vi "PBLV_Interface.vi"() -> ()   [LabVIEW 2013]
uses:
  <vilib>/Utility/error.llb/DialogTypeEnum.ctl
panel:
  in  "board_num":i32
  in  "change board":bool
  in  "# of Instructions":u32=4
  in  "Path to spinapi.dll":path=path "C:/SpinCore/SpinAPI/lib32/spinapi.dll"
  in  "start/restart":bool
  in  "load":bool
  in  "stop":bool
  in  "clock_freq (MHz)":dbl=100.0
  in  "Instructions":T1(array[cluster])=[{"Instruct Data"=0, "Op Code"=0, "Flags"=[FALSE, FALSE, FALSE, TRUE, FALSE, FALSE, FALSE, FALSE, FALSE, FALSE, FALSE, FALSE, FALSE, FALSE, FALSE, FALSE, FALSE, FALSE, FALSE, FALSE, FALSE, FALSE, FALSE, FALSE], "Comments"="", "Time (s)"=3e-05}, {"Instruct Data"=0, "Op Code"=0, "Flags"=[FALSE, TRUE, TRUE, FALSE, FALSE, FALSE, FALSE, FALSE, FALSE, FALSE, FALSE, FALSE, FALSE, FALSE, FALSE, FALSE, FALSE, FALSE, FALSE, FALSE, FALSE, FALSE, FALSE, FALSE], "Comments"="", "Time (s)"=0.5}, {"Instruct Data"=0, "Op Code"=0, "Flags"=[FALSE, FALSE, FALSE, TRUE, FALSE, FALSE, FALSE, FALSE, FALSE, FALSE, FALSE, FALSE, FALSE, FALSE, FALSE, FALSE, FALSE, FALSE, FALSE, FALSE, FALSE, FALSE, FALSE, FALSE], "Comments"="", "Time (s)"=3e-05}, {"Instruct Data"=0, "Op Code"=6, "Flags"=[FALSE, TRUE, TRUE, FALSE, FALSE, FALSE, FALSE, FALSE, FALSE, FALSE, FALSE, FALSE, FALSE, FALSE, FALSE, FALSE, FALSE, FALSE, FALSE, FALSE, FALSE, FALSE, FALSE, FALSE], "Comments"="", "Time (s)"=0.5}, {"Instruct Data"=0, "Op Code"=0, "Flags"=[TRUE, TRUE, TRUE, FALSE, FALSE, FALSE, FALSE, FALSE, FALSE, FALSE, FALSE, FALSE, FALSE, FALSE, FALSE, FALSE, FALSE, FALSE, FALSE, FALSE, FALSE, FALSE, FALSE, FALSE], "Comments"="", "Time (s)"=1.0}, {"Instruct Data"=0, "Op Code"=6, "Flags"=[FALSE, TRUE, TRUE, FALSE, FALSE, FALSE, FALSE, FALSE, FALSE, FALSE, FALSE, FALSE, FALSE, FALSE, FALSE, FALSE, FALSE, FALSE, FALSE, FALSE, FALSE, FALSE, FALSE, FALSE], "Comments"="", "Time (s)"=0.0015}] {"Time (s)" format="%.3p"; "Op Code" items=["Continue", "Stop", "Loop", "End Loop", "JSR", "RTS", "Branch", "Long Delay", "Wait"]}
  # "LabVIEW PulseBlaster Extension\nPulseBlaster Interface\nSpinCore Technologies, Inc.\nwww.spincore.com"
  # "Caution:    \n            After pressing STOP,\n            all output bits may \nmaintain their final state."
  # "1"
  # "2"
  # "3"
  # "4"
  # "5"
  # "6"
  # "7"
  # "8"
  # "9"
  # "10"
  # "11"
  # "12"
  # "13"
  # "14"
  # "15"
  # "16"
  # "17"
  # "18"
  # "19"
  # "20"
  # "21"
  # "22"
  # "23"
  # "24"
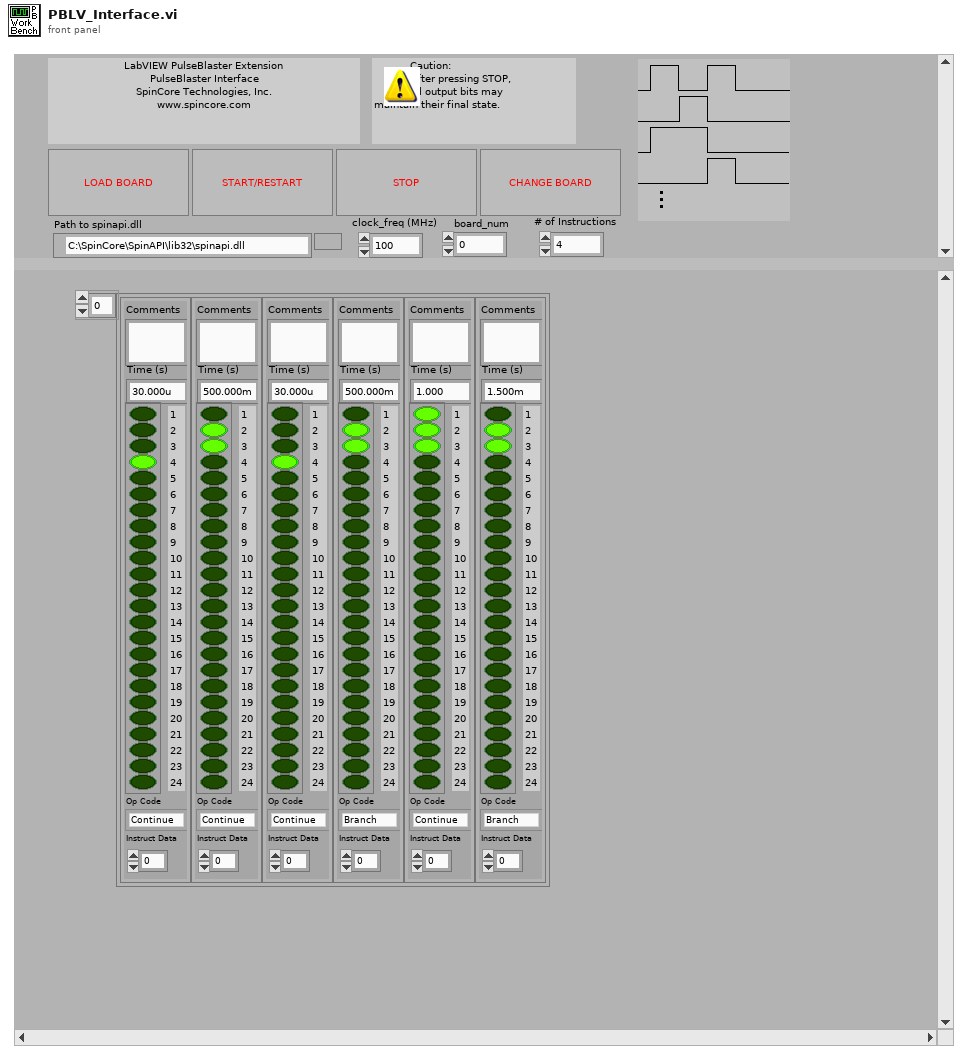
[diagram p1: front panel]
types:
  T1 = cluster{"Instruct Data":i32, "Op Code":i32, "Flags":bool[], "Comments":string, "Time (s)":dbl}[]
  T2 = typedef "DialogTypeEnum.ctl" = enum16{"no dialog", "OK message", "continue or stop message", "auto error handling dialog", "OK message + warnings", "continue/stop + warnings"}
  T3 = enum16{"Pulse Program", "Frequency Registers", "TX Phase Registers", "RX Phase Registers"}
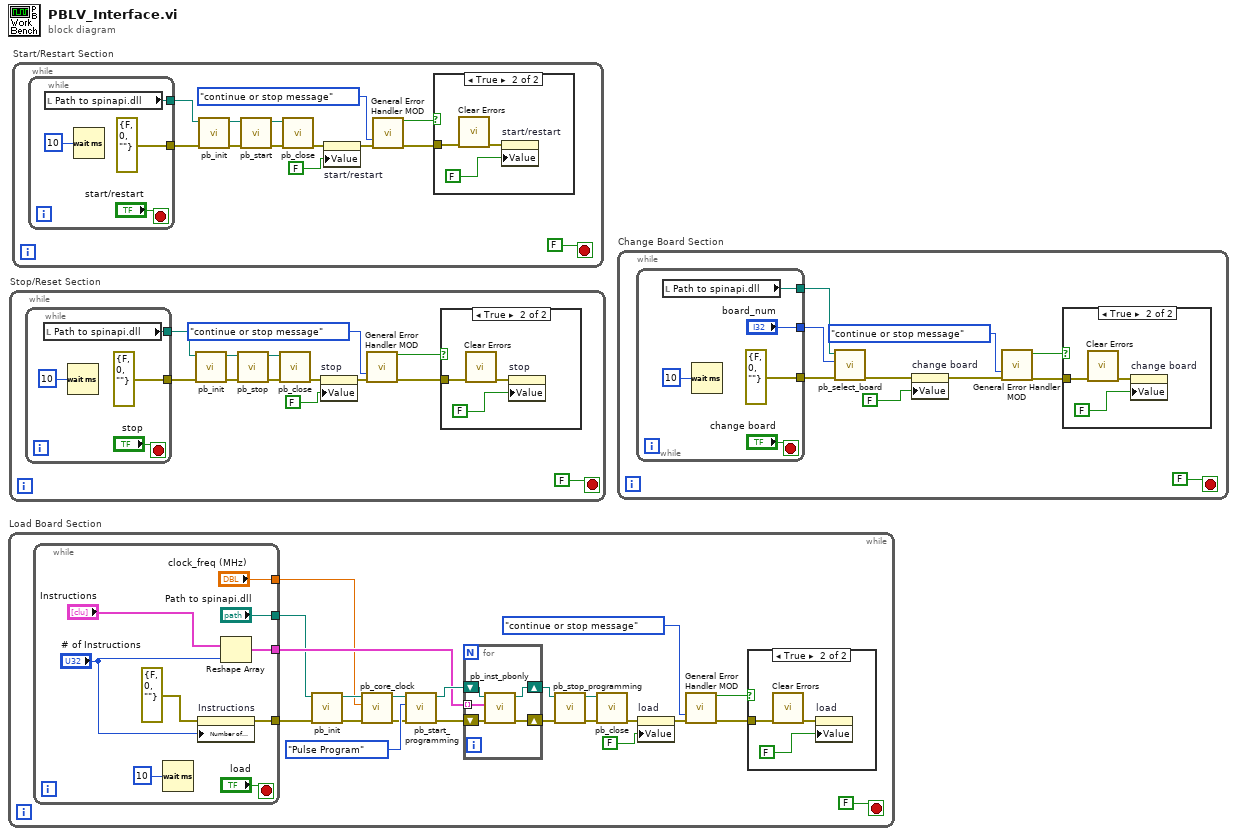
[diagram p0: block diagram]
diagram:
  n1 = while "Load Board Section" {
    stop <- FALSE stop-if-true
    n2 = while {
      tunnel: [w35] -> w17
      tunnel: [w36] -> w19
      tunnel: ["Path to spinapi.dll"] -> w2
      tunnel: ["clock_freq (MHz)"] -> w1
      stop <- "load" stop-if-true
      n3 = Wait (ms)(milliseconds to wait=u32 10) -> ()  [unwired: 1 out]
      n4 = property on="Instructions" class="Arr (strict)"(error in=errorcluster {"status"=FALSE, "code"=0, "source"=""} ("error in (no error)"), "Number of Columns"="# of Instructions") -> (error out=w35:errorcluster)  [unwired: 1 in, 1 out]
      n5 = Reshape Array("Instructions", "# of Instructions") -> (w36:T1)
    }
    n6 = call "pb_init.vi"("error in (no error)"=w17, "path in"=w2) -> ("error out"=w4:errorcluster, "path out"=w6:path)  [unwired: 2 in, 6 out]
    n7 = call "pb_core_clock.vi"("error in (no error)"=w4, "clock_freq (MHz)"=w1, "path in"=w6) -> ("error out"=w3:errorcluster, "path out"=w5:path)  [unwired: 7 in]
    n8 = call "pb_start_programming.vi"("error in (no error)"=w3, "Device"=T3."Pulse Program", "path in"=w5) -> ("error out"=w15:errorcluster, "path out"=w22:path)  [unwired: 1 in, 6 out]
    n9 = for {
      tunnel: w19 -> [w27] mode=indexing
      shift-right: [w29] -> w18
      shift-left: w22 -> [w30]
      shift-right: [w26] -> w14
      shift-left: w15 -> [w28]
      n10 = call "pb_inst_pbonly.vi"("error in (no error)"=w28, "PB Instruction"=w27, "path in"=w30) -> ("error out"=w26:errorcluster, "path out"=w29:path)  [unwired: 2 in, 5 out]
    }
    n11 = call "pb_stop_programming.vi"("error in (no error)"=w14, "path in"=w18) -> ("error out"=w13:errorcluster, "path out"=w21:path)  [unwired: 1 in, 7 out]
    n12 = call "pb_close.vi"("error in (no error)"=w13, "path in"=w21) -> ("error out"=w11:errorcluster)  [unwired: 9 out]
    n13 = property on="load" class="Bool (strict)"(error in=w11, "Value"=FALSE ("load")) -> (error out=w10:errorcluster)  [unwired: 1 in, 1 out]
    n14 = call "General Error Handler MOD.vi"("type of dialog (OK msg:1)"=DialogTypeEnum."continue or stop message", "error in (no error)"=w10) -> ("STOP?"=w7:bool, "error out"=w8:errorcluster)  [unwired: 12 out]
    n15 = case shown="True" w7 {
      tunnel: w8 -> [_ w25]
      frame False {
      }
      frame True {
        n16 = call <vilib>:"Clear Errors.vi"("error in (no error)"=w25) -> ("error out"=w23:errorcluster)  [unwired: 6 out]
        n17 = property on="load" class="Bool (strict)"(error in=w23, "Value"=FALSE ("Waiting for Data Acquisition")) -> ()  [unwired: 1 in, 2 out]
      }
    }
  }
  n18 = while "Stop/Reset Section" {
    stop <- FALSE stop-if-true
    n19 = while {
      tunnel: [errorcluster {"status"=FALSE, "code"=0, "source"=""} ("error in (no error)")] -> w49
      tunnel: [w56] -> w40
      stop <- "stop" stop-if-true
      n20 = local read "Path to spinapi.dll"() -> (w56:path)
      n21 = Wait (ms)(milliseconds to wait=u32 10) -> ()  [unwired: 1 out]
    }
    n22 = call "pb_init.vi"("error in (no error)"=w49, "path in"=w40) -> ("error out"=w48:errorcluster, "path out"=w51:path)  [unwired: 1 in, 7 out]
    n23 = call "pb_stop.vi"("error in (no error)"=w48, "path in"=w51) -> ("error out"=w47:errorcluster, "path out"=w52:path)  [unwired: 8 out]
    n24 = call "pb_close.vi"("error in (no error)"=w47, "path in"=w52) -> ("error out"=w46:errorcluster)  [unwired: 9 out]
    n25 = property on="stop" class="Bool (strict)"(error in=w46, "Value"=FALSE ("stop")) -> (error out=w45:errorcluster)  [unwired: 1 in, 1 out]
    n26 = call "General Error Handler MOD.vi"("type of dialog (OK msg:1)"=DialogTypeEnum."continue or stop message", "error in (no error)"=w45) -> ("STOP?"=w42:bool, "error out"=w41:errorcluster)  [unwired: 12 out]
    n27 = case shown="True" w42 {
      tunnel: w41 -> [_ w55]
      frame False {
      }
      frame True {
        n28 = call <vilib>:"Clear Errors.vi"("error in (no error)"=w55) -> ("error out"=w53:errorcluster)  [unwired: 6 out]
        n29 = property on="stop" class="Bool (strict)"(error in=w53, "Value"=FALSE ("Waiting for Data Acquisition")) -> ()  [unwired: 1 in, 2 out]
      }
    }
  }
  n30 = while "Start/Restart Section" {
    stop <- FALSE stop-if-true
    n31 = while {
      tunnel: [errorcluster {"status"=FALSE, "code"=0, "source"=""} ("error in (no error)")] -> w69
      tunnel: [w76] -> w60
      stop <- "start/restart" stop-if-true
      n32 = local read "Path to spinapi.dll"() -> (w76:path)
      n33 = Wait (ms)(milliseconds to wait=u32 10) -> ()  [unwired: 1 out]
    }
    n34 = call "pb_init.vi"("error in (no error)"=w69, "path in"=w60) -> ("error out"=w68:errorcluster, "path out"=w71:path)  [unwired: 1 in, 7 out]
    n35 = call "pb_start.vi"("error in (no error)"=w68, "path in"=w71) -> ("error out"=w67:errorcluster, "path out"=w72:path)  [unwired: 1 in, 7 out]
    n36 = call "pb_close.vi"("error in (no error)"=w67, "path in"=w72) -> ("error out"=w66:errorcluster)  [unwired: 9 out]
    n37 = property on="start/restart" class="Bool (strict)"(error in=w66, "Value"=FALSE ("start/restart")) -> (error out=w65:errorcluster)  [unwired: 1 in, 1 out]
    n38 = call "General Error Handler MOD.vi"("type of dialog (OK msg:1)"=DialogTypeEnum."continue or stop message", "error in (no error)"=w65) -> ("STOP?"=w62:bool, "error out"=w61:errorcluster)  [unwired: 12 out]
    n39 = case shown="True" w62 {
      tunnel: w61 -> [_ w75]
      frame False {
      }
      frame True {
        n40 = call <vilib>:"Clear Errors.vi"("error in (no error)"=w75) -> ("error out"=w73:errorcluster)  [unwired: 6 out]
        n41 = property on="start/restart" class="Bool (strict)"(error in=w73, "Value"=FALSE ("Waiting for Data Acquisition")) -> ()  [unwired: 1 in, 2 out]
      }
    }
  }
  n42 = while "Change Board Section" {
    stop <- FALSE stop-if-true
    n43 = while {
      tunnel: [errorcluster {"status"=FALSE, "code"=0, "source"=""} ("error in (no error)")] -> w89
      tunnel: ["board_num"] -> w88
      tunnel: [w93] -> w80
      stop <- "change board" stop-if-true
      n44 = local read "Path to spinapi.dll"() -> (w93:path)
      n45 = Wait (ms)(milliseconds to wait=u32 10) -> ()  [unwired: 1 out]
    }
    n46 = call "pb_select_board.vi"("error in (no error)"=w89, "board_num"=w88, "path in"=w80) -> ("error out"=w86:errorcluster)  [unwired: 8 out]
    n47 = property on="change board" class="Bool (strict)"(error in=w86, "Value"=FALSE ("change board")) -> (error out=w85:errorcluster)  [unwired: 1 in, 1 out]
    n48 = call "General Error Handler MOD.vi"("type of dialog (OK msg:1)"=DialogTypeEnum."continue or stop message", "error in (no error)"=w85) -> ("STOP?"=w82:bool, "error out"=w81:errorcluster)  [unwired: 12 out]
    n49 = case shown="True" w82 {
      tunnel: w81 -> [_ w92]
      frame False {
      }
      frame True {
        n50 = call <vilib>:"Clear Errors.vi"("error in (no error)"=w92) -> ("error out"=w90:errorcluster)  [unwired: 6 out]
        n51 = property on="change board" class="Bool (strict)"(error in=w90, "Value"=FALSE ("Waiting for Data Acquisition")) -> ()  [unwired: 1 in, 2 out]
      }
    }
  }
